vi "Digital Write 1 Chan.vi"(8 "Error In":errorcluster, 9 "Output Value":bool, 10 "DO Channel":u8, 11 "LINX Resource":T1) -> (0 "Error Out":errorcluster, 3 "LINX Resource":T1)   [LabVIEW 2013, in "LVH-LINX.lvlib"]
doc: "Write a value to the specified digital output channel."
uses:
  <vilib>/LabVIEW Hacker/LINX/LVH-LINX.lvlib
  <vilib>/LabVIEW Hacker/LINX/Private/Type Defs/LINX Ref.ctl
  <vilib>/LabVIEW Hacker/LINX/Private/Type Defs/Platform.ctl
  <vilib>/LabVIEW Hacker/LINX/Private/Type Defs/Interface.ctl
  <vilib>/LabVIEW Hacker/LINX/Private/Device/Type Defs/LINX Device Config.ctl
  <vilib>/LabVIEW Hacker/LINX/Private/Device/Type Defs/TCP Config.ctl
  <vilib>/LabVIEW Hacker/LINX/Private/Type Defs/Device Family.ctl
  <vilib>/LabVIEW Hacker/LINX/Private/Device/Device.lvlib
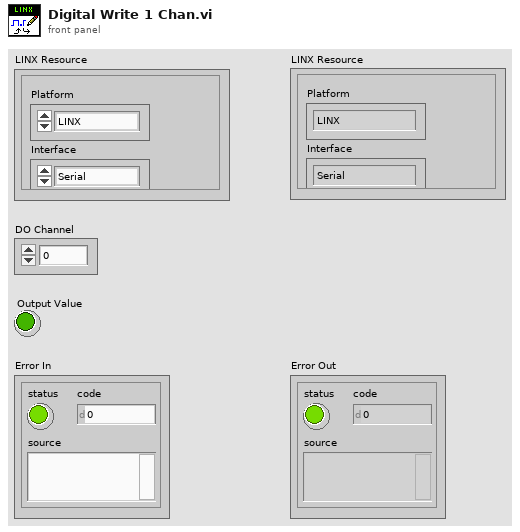
[diagram p1: front panel]
types:
  T1 = typedef "LVH-LINX.lvlib/LINX Ref.ctl" = cluster{"Platform":T2, "Interface":T3, "LINX Device Config":T4}
  T2 = typedef "LVH-LINX.lvlib/Platform.ctl" = enum16{"LINX", "myRIO"}
  T3 = typedef "LVH-LINX.lvlib/Interface.ctl" = enum16{"Serial", "TCP"}
  T4 = typedef "LVH-LINX.lvlib/Device.lvlib/LINX Device Config.ctl" = cluster{"Interface":T3, "COM Port":refnum<visa-resource-name>, "TCP Configuration":T5, "Device Family":T6, "Device ID":u8, "Device Name":string, "TCP Ref":refnum<k5>}
  T5 = typedef "LVH-LINX.lvlib/Device.lvlib/TCP Config.ctl" = cluster{"IP Address":string, "Port":u16}
  T6 = typedef "LVH-LINX.lvlib/Device Family.ctl" = enum8{"National Instruments", "Digilent", "Arduino"}
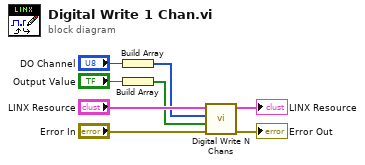
[diagram p0: block diagram]
diagram:
  n1 = Build Array("DO Channel") -> (w1:u8[])
  n2 = Build Array("Output Value") -> (w2:bool[])
  n3 = call <vilib>:"Digital Write N Chans.vi"("Error In"="Error In", "Values"=w2, "DO Channels"=w1, "LINX Resource"="LINX Resource") -> ("Error Out"=→"Error Out":errorcluster, "LINX Resource"=→"LINX Resource":T1)  [unwired: 6 in]
